vi "Enable Binning Strobe.vi"(8 "error in (no error)":errorcluster, 10 "Enable Binning Strobe (F: Disable)":bool, 11 "VISA resource name":refnum<visa-resource-name>) -> (0 "error out":errorcluster, 3 "VISA resource name out":refnum<visa-resource-name>)   [LabVIEW 2020, in "Keithley 6517.lvlib"]
doc: "Controls the binning strobe for CALC 3.\n\n<B>Note:</B>\nThis VI is <B>NOT</B> compatible with model <B>6514</B>."
uses:
  <instrlib>/Keithley 6517/Keithley 6517.lvlib
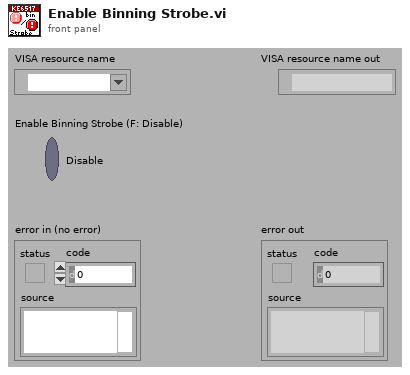
[diagram p1: front panel]
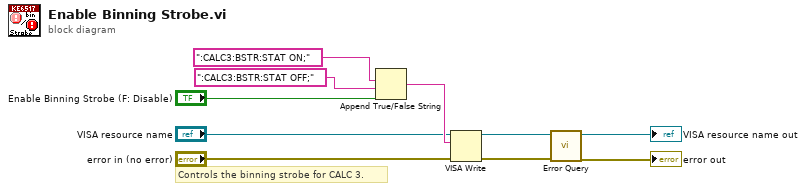
[diagram p0: block diagram]
diagram:
  # "Controls the binning strobe for CALC 3."
  n1 = Append True/False String(1:"Enable Binning Strobe (F: Disable)", 2:":CALC3:BSTR:STAT OFF;", 3:":CALC3:BSTR:STAT ON;") -> (0:w7:string)  [unwired: 1 in]
  n2 = VISA Write(VISA resource name="VISA resource name", write buffer=w7, error in (no error)="error in (no error)") -> (VISA resource name out=w4:refnum<visa-resource-name>, error out=w3:errorcluster)  [unwired: 1 out]
  n3 = call <instrlib>:"Error Query.vi"("error in (no error)"=w3, "VISA resource name"=w4) -> ("error out"=→"error out":errorcluster, "VISA resource name out"=→"VISA resource name out":refnum<visa-resource-name>)  [unwired: 6 in, 2 out]
